vi "Unit Test.vi"() -> ()   [LabVIEW 2018]
uses:
  PPLs/Optical Power Meter/Optical Power Meter.lvlibp/Custom Controls/Channel List.ctl
  2936r.lvclass
  PPLs/Optical Power Meter/Optical Power Meter.lvlibp/Custom Controls/Measurement Mode.ctl
  C:/Projects/LabVIEW/Built/Optical Power Meter/2936R/Required library/PowerMeterCommands.dll
  Required library/PowerMeterCommands.dll
  PPLs/Optical Power Meter/Optical Power Meter.lvlibp
panel:
  in  "Auto Range":bool
  in  "Range Level":u32
  in  "Wavelength (nm)":dbl=1550.0 format="%#_13g"
  in  "Channel":T1
  out "Average Power":dbl
  out "Power":dbl
  out "Measured Power":dbl[](array[numeric])
  in  "error in":errorcluster
  out "error out":errorcluster
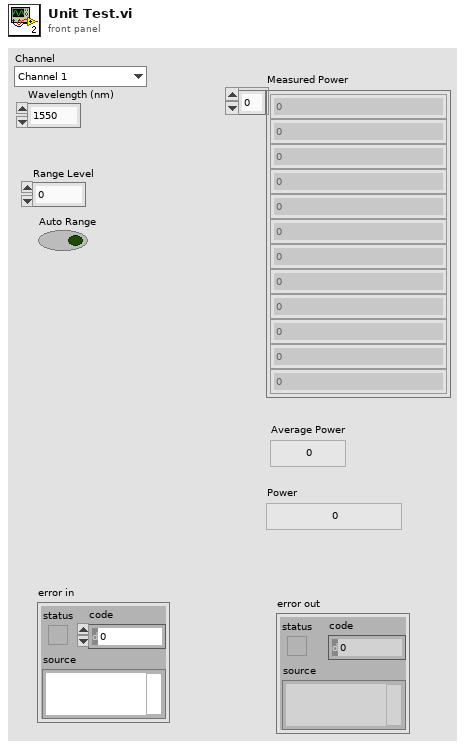
[diagram p1: front panel]
types:
  T1 = typedef "Optical Power Meter.lvlibp/Channel List.ctl" = enum16{"Channel 1", "Channel 2", "Channel 3", "Channel 4"}
  T2 = typedef "Optical Power Meter.lvlibp/Measurement Mode.ctl" = enum16{"CW Continuous", "CW Single", "CW Integrate", "PK-PK Continuous", "PK-PK Single", "RMS"}
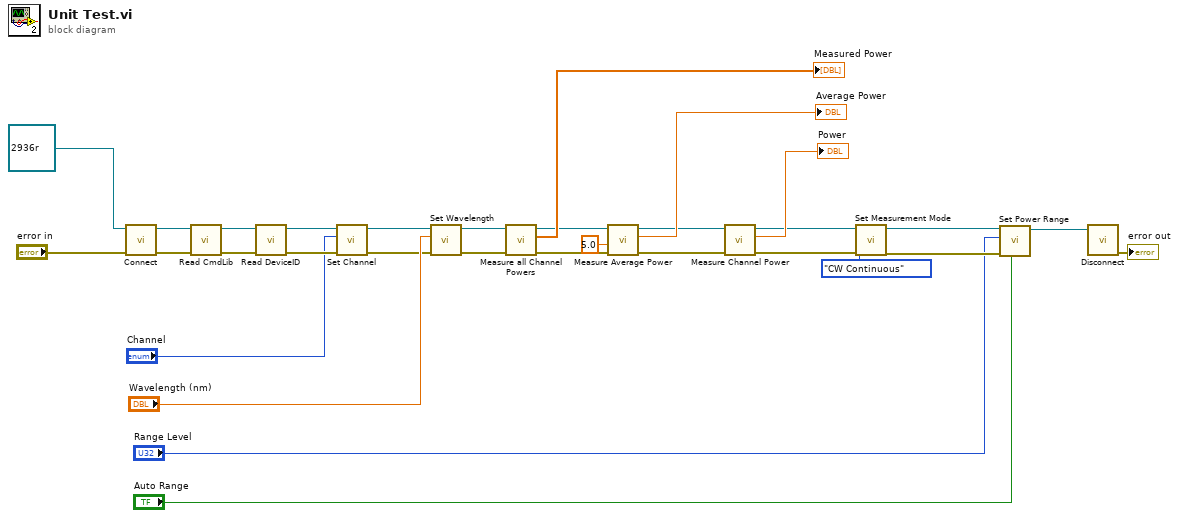
[diagram p0: block diagram]
diagram:
  n1 = call-dynamic "Connect.vi"("error in"="error in", "2936r in"=refnum<class "2936r.lvclass"> refnum) -> ("error out"=w27:errorcluster, "2936r out"=w28:refnum<class "2936r.lvclass">)  [unwired: 8 in]
  n2 = call "Read CmdLib.vi"("error in (no error)"=w27, "2936r in"=w28) -> ("error out"=w25:errorcluster, "2936r out"=w26:refnum<class "2936r.lvclass">)  [unwired: 7 in, 1 out]
  n3 = call "Read DeviceID.vi"("error in (no error)"=w25, "2936r in"=w26) -> ("error out"=w10:errorcluster, "2936r out"=w11:refnum<class "2936r.lvclass">)  [unwired: 7 in, 1 out]
  n4 = call-dynamic "Set Channel.vi"("error in (no error)"=w10, "Channel"="Channel", "2936r in"=w11) -> ("error out"=w8:errorcluster, "2936r out"=w9:refnum<class "2936r.lvclass">)  [unwired: 7 in]
  n5 = call-dynamic "Set Wavelength.vi"("error in"=w8, "Wavelength (nm)"="Wavelength (nm)", "2936r in"=w9) -> ("error out"=w12:errorcluster, "2936r out"=w13:refnum<class "2936r.lvclass">)  [unwired: 7 in]
  n6 = call-dynamic "Measure all Channel Powers.vi"("error in (no error)"=w12, "2936r in"=w13) -> ("error out"=w3:errorcluster, "Measured Power"=→"Measured Power":dbl[], "2936r out"=w5:refnum<class "2936r.lvclass">)  [unwired: 7 in]
  n7 = call-dynamic "Measure Average Power.vi"("error in"=w3, "# Samples in"=5.0, "2936r in"=w5) -> ("error out"=w2:errorcluster, "Average Power"=→"Average Power":dbl, "2936r out"=w4:refnum<class "2936r.lvclass">)  [unwired: 5 in, 1 out]
  n8 = call-dynamic "Measure Channel Power.vi"("error in"=w2, "2936r in"=w4) -> ("error out"=w20:errorcluster, "Power"=→"Power":dbl, "2936r out"=w21:refnum<class "2936r.lvclass">)  [unwired: 7 in]
  n9 = call-dynamic "Set Measurement Mode.vi"("error in (no error)"=w20, "Measurement Mode"=Measurement_Mode."CW Continuous", "2936r in"=w21) -> ("error out"=w16:errorcluster, "2936r out"=w18:refnum<class "2936r.lvclass">)  [unwired: 7 in]
  n10 = call-dynamic "Set Power Range.vi"("Auto Range"="Auto Range", "error in (no error)"=w16, "Power Level"="Range Level", "2936r in"=w18) -> ("2936r out"=w17:refnum<class "2936r.lvclass">)  [unwired: 6 in, 1 out]
  n11 = call-dynamic "Disconnect.vi"("2936r in"=w17) -> ("error out"=→"error out":errorcluster)  [unwired: 9 in, 1 out]
